vi "DT_Triangle Manager_Get Oppo Point_in Ghost.vi"(9 "point idx":i32, 10 "triangle":i32, 11 "Triangles":i32[][](array[numeric])) -> (2 "opposite point idx":i32)   [LabVIEW 2017, in "NI_AAL_Geometry.lvlib"]
uses:
  <vilib>/Analysis/NI_AAL_Geometry.lvlib
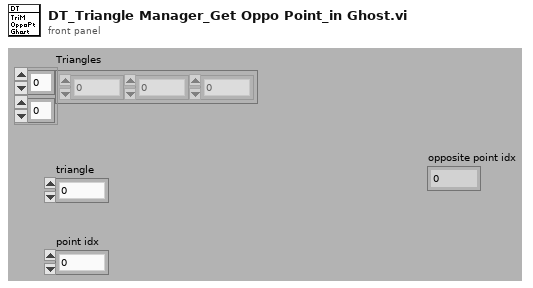
[diagram p1: front panel]
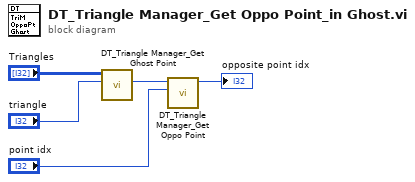
[diagram p0: block diagram]
diagram:
  n1 = call <vilib>:"DT_Triangle Manager_Get Ghost Point.vi"("triangle"="triangle", "Triangles In"="Triangles") -> ("ghost point idx"=w3:i32)  [unwired: 9 out]
  n2 = call <vilib>:"DT_Triangle Manager_Get Oppo Point.vi"("point idx 2"="point idx", "point idx 1"=w3) -> ("oppo point idx"=→"opposite point idx":i32)  [unwired: 9 out]
